vi "Get list of FOM initialization steps.vi"() -> (3 "init steps":string[](array[string]))   [LabVIEW 2019, in "HLA Custom Device Engine.lvlib"]
uses:
  HLA Custom Device Engine.lvlib
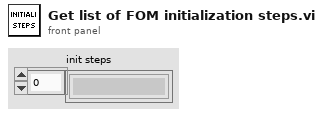
[diagram p1: front panel]
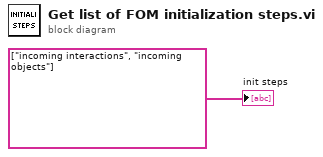
[diagram p0: block diagram]
diagram:
  "init steps" <- string[] ["incoming interactions", "incoming objects"] ("init steps")
